vi "GroundPassWrapper.vi"(7 "State":T1=enum."Pass", 8 "error in":errorcluster) -> (0 "error out":errorcluster)   [LabVIEW 2013]
doc: "Wrapper for ground pass. It has the following actions:\n-Pass: sets the clapper to out, the roller pneumatic to middle, and the roller motor to reverse.\n-Stop: sets the clapper to in and the roller motor to off."
uses:
  PassState.ctl
  DoubleSolenoidAction.ctl
  RollerAction.ctl
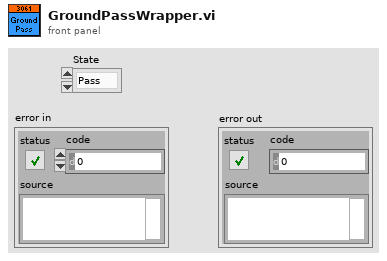
[diagram p1: front panel]
types:
  T1 = typedef "PassState.ctl" = enum16{"Stop", "Pass"}
  T2 = typedef "DoubleSolenoidAction.ctl" = enum16{"Init", "Middle", "In", "Out"}
  T3 = typedef "RollerAction.ctl" = enum16{"Init", "Off", "Forward", "Reverse"}
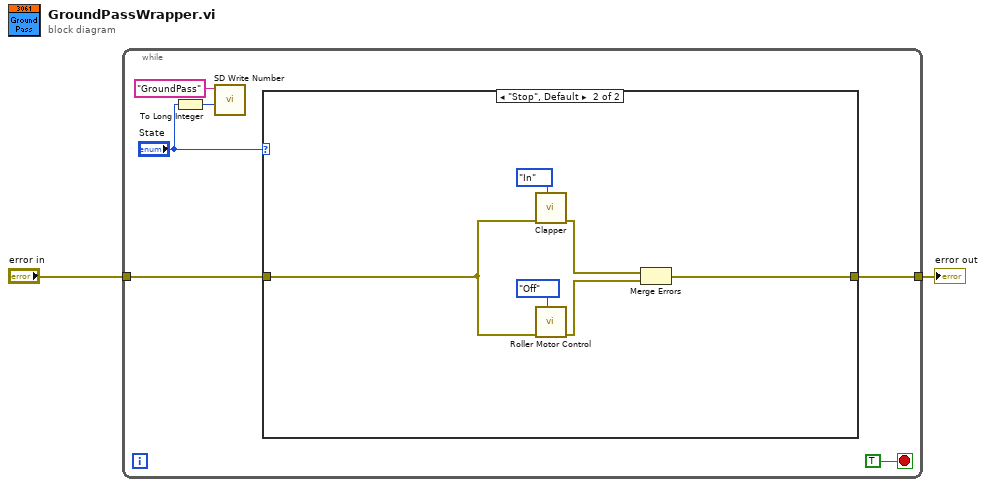
[diagram p0: block diagram]
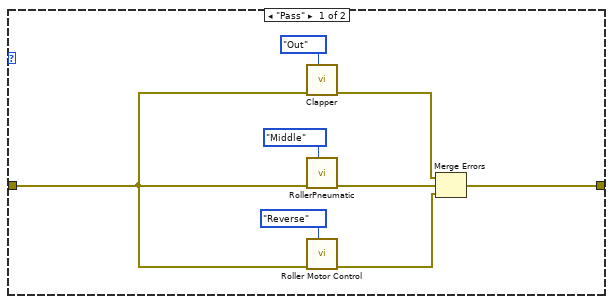
[diagram p2: hidden frame]
diagram:
  n1 = while {
    tunnel: "error in" -> [w7]
    tunnel: [w6] -> w1
    stop <- TRUE stop-if-true
    n2 = To Long Integer(number="State") -> (32bit integer=w4:i32)
    n3 = call <vilib>:"SD Write Number.vi"("Numeric"=w4, "Name"="GroundPass") -> ()  [unwired: 8 in, 2 out]
    n4 = case shown="\"Stop\", Default" "State" {
      tunnel: w7 -> [w13 w20]
      tunnel: [w9 w17] -> w6
      frame "Pass" {
        n5 = call "Clapper.vi"("State"=DoubleSolenoidAction."Out", "Error in"=w13) -> ("Error out"=w12:errorcluster)  [unwired: 9 in]
        n6 = call "RollerPneumatic.vi"("State"=DoubleSolenoidAction."Middle", "Error in"=w13) -> ("Error out"=w11:errorcluster)  [unwired: 9 in]
        n7 = call "Roller Motor Control.vi"("Action"=RollerAction."Reverse", "Error in"=w13) -> ("Error out"=w10:errorcluster)  [unwired: 9 in]
        n8 = Merge Errors(w12, w11, w10) -> (w9:errorcluster)
      }
      frame "Stop", Default {
        n9 = call "Clapper.vi"("State"=DoubleSolenoidAction."In", "Error in"=w20) -> ("Error out"=w19:errorcluster)  [unwired: 9 in]
        n10 = call "Roller Motor Control.vi"("Action"=RollerAction."Off", "Error in"=w20) -> ("Error out"=w18:errorcluster)  [unwired: 9 in]
        n11 = Merge Errors(w19, w18) -> (w17:errorcluster)
      }
    }
  }
  "error out" <- w1
